vi "Instrument.Oxford1820.sendMessageToProcess.vi"(6 "ID":string, 8 "error in (no error)":errorcluster, 9 "Data":variant, 10 "Command":string, 11 "Instrument.Oxford1820":refnum<class "Instrument.Oxford1820.lvclass">) -> (0 "error out":errorcluster, 3 "Instrument.Oxford1820 out":refnum<class "Instrument.Oxford1820.lvclass">)   [LabVIEW 2019, in "Instrument.Oxford1820.lvclass"]
doc: "---------------------------------------------------------------\nJKI State Machine Objects™\nhttp://jki.net/state-machine-objects/\nCopyright (C) 2005-2015, JKI <info@jki.net>\nALL RIGHTS RESERVEDJKI State Machine Objects (SMO) 1.0.0.4\nJKI - JKI\nCopyright (c) 2015, JKI"
uses:
  Instrument.Oxford1820.lvclass
  Typedefs/PrivateEvents--Instrument.Oxford1820.MessageToProcess.ctl
  <userlib>/LevyLab/Instrument Framework/SMOs/RemoteControl/Typedefs/Message--Cluster.ctl
  Instrument.Oxford1820.lvclass/Instrument.Oxford1820.ctl
  <userlib>/LevyLab/Instrument Framework/SMOs/RemoteControl/RemoteControl.lvclass
panel:
  # "For instructions on how to use the JKI State Machine Objects, examples and video tutorials, visit:\nhttp://jki.net/state-machine-objects/\n\nJKI State Machine Objects™\nhttp://jki.net/state-machine-objects/\nCopyright (C) 2005-2015, JKI <info@jki.net>\nALL RIGHTS RESERVED"
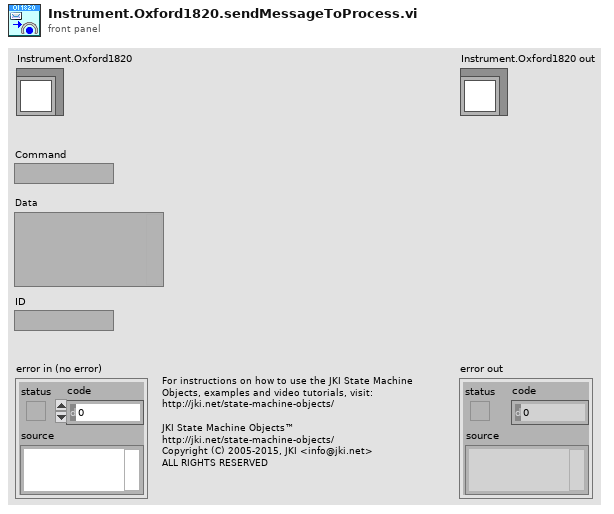
[diagram p1: front panel]
types:
  T1 = typedef "Instrument.Oxford1820.lvclass/PrivateEvents--Instrument.Oxford1820.MessageToProcess.ctl" = cluster{"Message":T2}
  T2 = typedef "RemoteControl.lvclass/Message--Cluster.ctl" = cluster{"Command":string, "Data":variant, "ID":string}
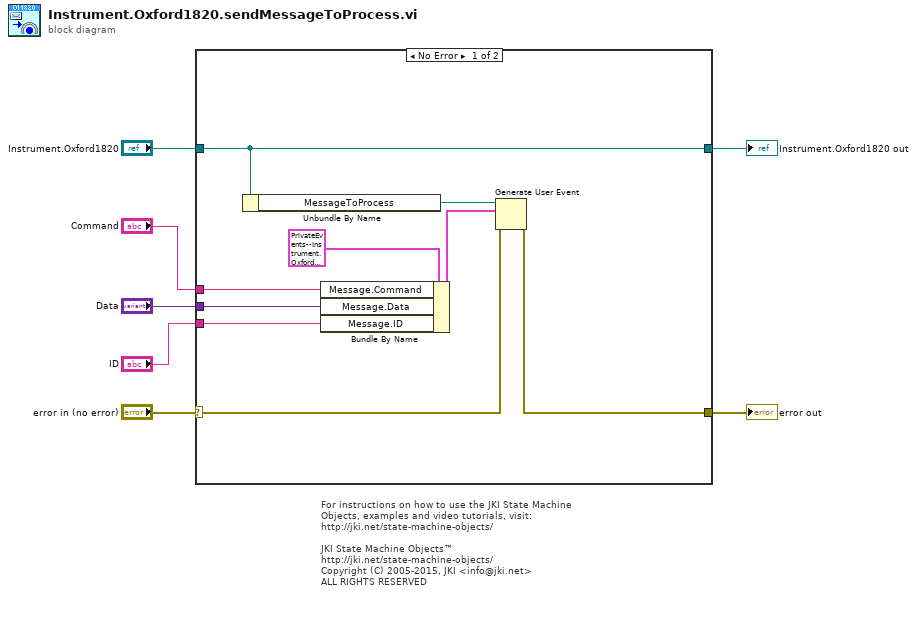
[diagram p0: block diagram]
diagram:
  # "For instructions on how to use the JKI State Machine Objects, examples and video tutorials, visit:\nhttp://jki.net/state-machine-objects/\n\nJKI State Machine Objects™\nhttp://jki.net/state-machine-objects/\nCopyright (C) 2005-2015, JKI <info@jki.net>\nALL RIGHTS RESERVED"
  n1 = case shown="No Error" "error in (no error)" {
    selector: "error in (no error)" -> [w16 w18]
    tunnel: [w14 w18] -> w6
    tunnel: [w13 w17] -> w7
    tunnel: "Instrument.Oxford1820" -> [w13 w17]
    tunnel: "Command" -> [w10 _]
    tunnel: "Data" -> [w9 _]
    tunnel: "ID" -> [w8 _]
    frame No Error {
      n2 = Unbundle By Name(w13) -> ("MessageToProcess"=w15:refnum<user-event>)
      n3 = Bundle By Name(cluster=T1 {"Message"={"Command"="", "Data"=variant(string ""), "ID"=""}} ("event data"), "Message.Command"=w10, "Message.Data"=w9, "Message.ID"=w8) -> (w11:T1)
      n4 = Generate User Event(user event=w15, event data cluster=w11, error in=w16) -> (error out=w14:errorcluster)  [unwired: 1 in, 1 out]
    }
    frame Error {
    }
  }
  "error out" <- w6
  "Instrument.Oxford1820 out" <- w7
